vi "Read Device Identification.vi"(8 "error in":errorcluster, 9 "read device ID code":T2, 10 "object ID":u8, 11 "Modbus instance in":refnum<class "Modbus API.lvclass">) -> (0 "error out":errorcluster, 2 "objects":T1[](array[typedef]) {"Object ID" format="%x"}, 3 "Modbus instance out":refnum<class "Modbus API.lvclass">)   [LabVIEW 2021, in "Modbus API.lvclass"]
doc: "Reads Modbus object information stored on the device. This can include basic information, like manufacturer, additional standard items, or model-specific extended items. This function may take a large amount of time to execute, as it requires the transfer of a large quantity of binary data. Even on TCP/IP, this function is limited by the maximum defined size of a Modbus protocol data unit."
uses:
  Modbus API.lvclass
  Master Function Definition/Read Device ID code.ctl
  Data Model/Identification Parameters.ctl
  Data Model/Device Data Model.lvclass
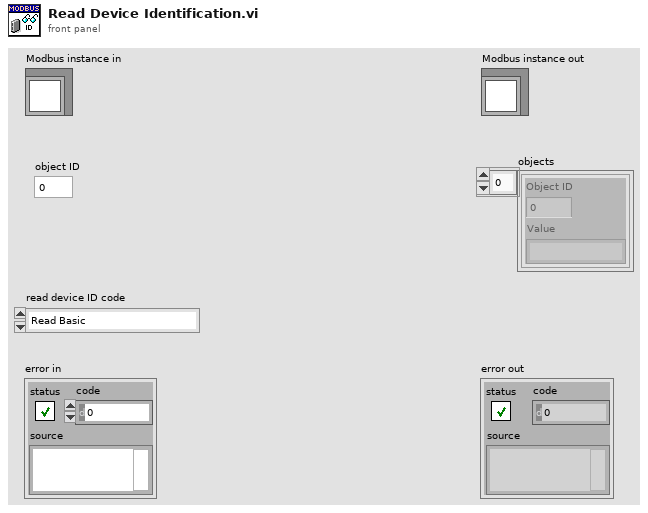
[diagram p1: front panel]
types:
  T1 = typedef "Device Data Model.lvclass/Identification Parameters.ctl" = cluster{"Object ID":u8, "Value":string}
  T2 = typedef "Device Data Model.lvclass/Read Device ID code.ctl" = enum8{"Read Basic", "Read Regular", "Read Extended", "Read Specific"}
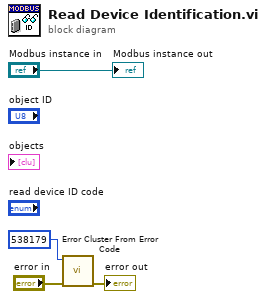
[diagram p0: block diagram]
diagram:
  n1 = call <vilib>:"Error Cluster From Error Code.vi"("error in (no error)"="error in", "error code (0)"=538179) -> ("error out"=→"error out":errorcluster)  [unwired: 7 in]
  "Modbus instance out" <- "Modbus instance in"
